vi "Error - Write TXT.vi"(7 "operation":T1(ring)=enum."replace or create", 8 "error in":errorcluster, 9 "text":string, 10 "filename.txt":string="error_log.txt", 11 "base path":path) -> (0 "error out":errorcluster)   [LabVIEW 2017]
doc: "This SubVI open or create a predefined txt file in certain directory"
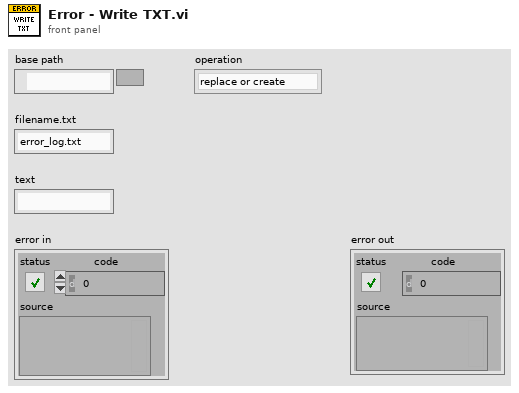
[diagram p1: front panel]
types:
  T1 = enum16{"open", "replace", "create", "open or create", "replace or create", "replace or create with confirmation"}
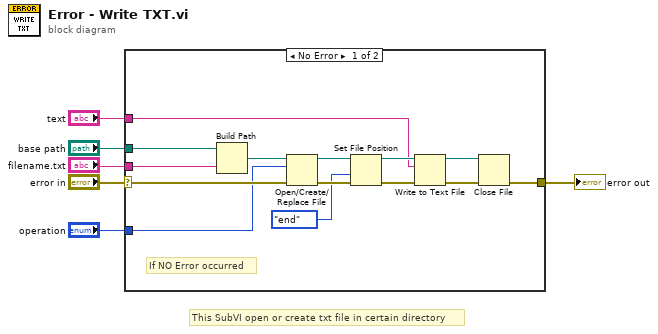
[diagram p0: block diagram]
diagram:
  # "This SubVI open or create txt file in certain directory"
  n1 = case shown="No Error" "error in" {
    selector: "error in" -> [w12 w21]
    tunnel: [w11 w21] -> w5
    tunnel: "filename.txt" -> [w10 _]
    tunnel: "base path" -> [w9 _]
    tunnel: "text" -> [w8 _]
    tunnel: "operation" -> [w7 _]
    frame No Error {
      # "If NO Error occurred"
      n2 = Build Path(base path=w9, name or relative path=w10) -> (appended path=w20:path)
      n3 = Open/Create/Replace File(file path (use dialog)=w20, error in=w12, operation (0:open)=w7) -> (refnum out=w19:refnum<file>, error out=w18:errorcluster)  [unwired: 3 in, 1 out]
      n4 = Set File Position(refnum=w19, from (0:start)=enum16{"start", "end", "current"}."end", error in=w18) -> (refnum out=w17:refnum<file>, error out=w16:errorcluster)  [unwired: 1 in]
      n5 = Write to Text File(file (use dialog)=w17, text=w8, error in=w16) -> (refnum out=w14:refnum<file>, error out=w15:errorcluster)  [unwired: 1 in, 1 out]
      n6 = Close File(refnum=w14, error in=w15) -> (error out=w11:errorcluster)  [unwired: 1 out]
    }
    frame Error {
      # "If any error occurred"
    }
  }
  "error out" <- w5
